vi "Default Configuration--constant.vi"() -> (3 "Default Configuration":T1)   [LabVIEW 2020, in "Performance Monitor UI.lvlib" / "Configuration.lvlib"]
doc: "This VI stores the default data to be saved in the config file, when application executes for the very first time, the file doesn't exist or the config file is corrupted.\n_____\nBased on DCFG Project Template 1.0.0.21.\n____\nPeloton Config 1.0.0.2\nCopyright (c) 2022, Peloton"
uses:
  Configuration.lvlib
  Configuration--cluster.ctl
  <vilib>/Utility/sysdir.llb/System Directory Type.ctl
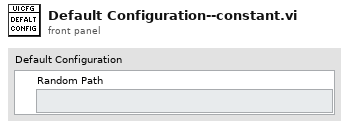
[diagram p1: front panel]
types:
  T1 = typedef "Performance Monitor UI.lvlib/Configuration.lvlib/Configuration--cluster.ctl" = cluster{"Random Path":path}
  T2 = typedef "System Directory Type.ctl" = i32
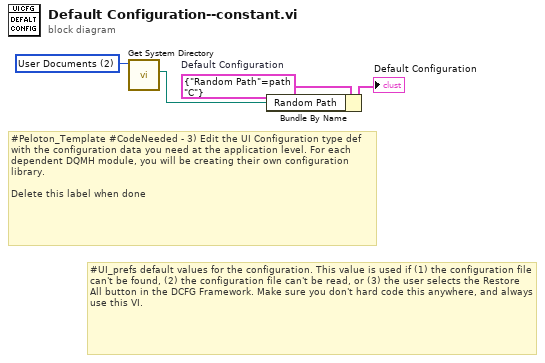
[diagram p0: block diagram]
diagram:
  w2 = T2 2 items=["User Home"=0, "User Desktop"=1, "User Documents"=2, "User Application Data"=3, "User Preferences"=4, "User Temporary"=5, "Public Documents"=6, "Public Application Data"=7, "Public Preferences"=8, "Public Cache"=13, "System Core Libraries"=9, "System Installed Libraries"=10, "Application Files"=11, "Boot Volume Root"=12] ("system directory type")
  w4 = T1 {"Random Path"=path "C:/"}  # Default Configuration
  # "#Peloton_Template #CodeNeeded - 3) Edit the UI Configuration type def with the configuration data you need at the application level. For each dependent DQMH module, you will be creating their own configuration library.\n\nDelete this label when done"
  # "#UI_prefs default values for the configuration. This value is used if (1) the configuration file can't be found, (2) the configuration file can't be read, or (3) the user selects the Restore All button in the DCFG Framework. Make sure you don't hard code this anywhere, and always use this VI."
  n1 = call <vilib>:"Get System Directory.vi"("system directory type"=w2) -> ("system directory"=w1:path)  [unwired: 10 in]
  n2 = Bundle By Name(cluster=w4, "Random Path"=w1) -> (→"Default Configuration":T1)
